vi "Waveform Channel Selection.vi"() -> ()   [LabVIEW 2015]
uses:
  NationalInstruments.VeriStand.SystemDefinitionAPI
  NationalInstruments.VeriStand.SystemStorage
  NationalInstruments.VeriStand
panel:
  in  "Commit Waveforms":bool
  in  "path":path=path "C:/Users/Public/Documents/National Instruments/NI VeriStand 2015/Examples/Stimulus Profile/Engine Demo/Engine Demo.nivssdf"
  in  "Stop Button":bool
  in  "Waveforms to Process":i32(listbox)
  in  "Available Unused Waveforms":i32(listbox)
  in  "Waveform Task":u16(ring) items=["Waveform1"=11, "Waveform2"=15]
  in  "Remove Channel":bool
  in  "Add Channel":bool
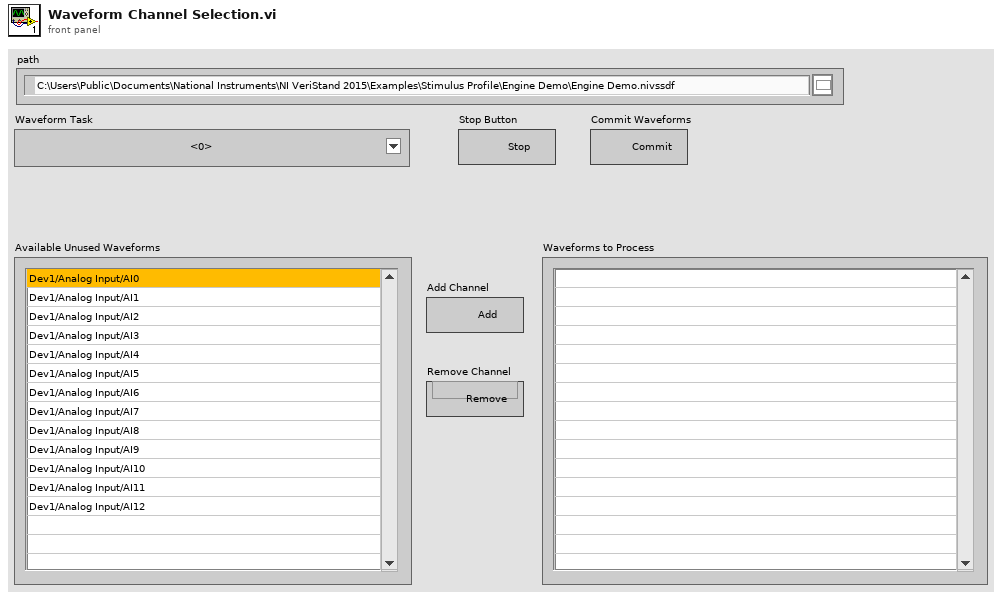
[diagram p1: front panel]
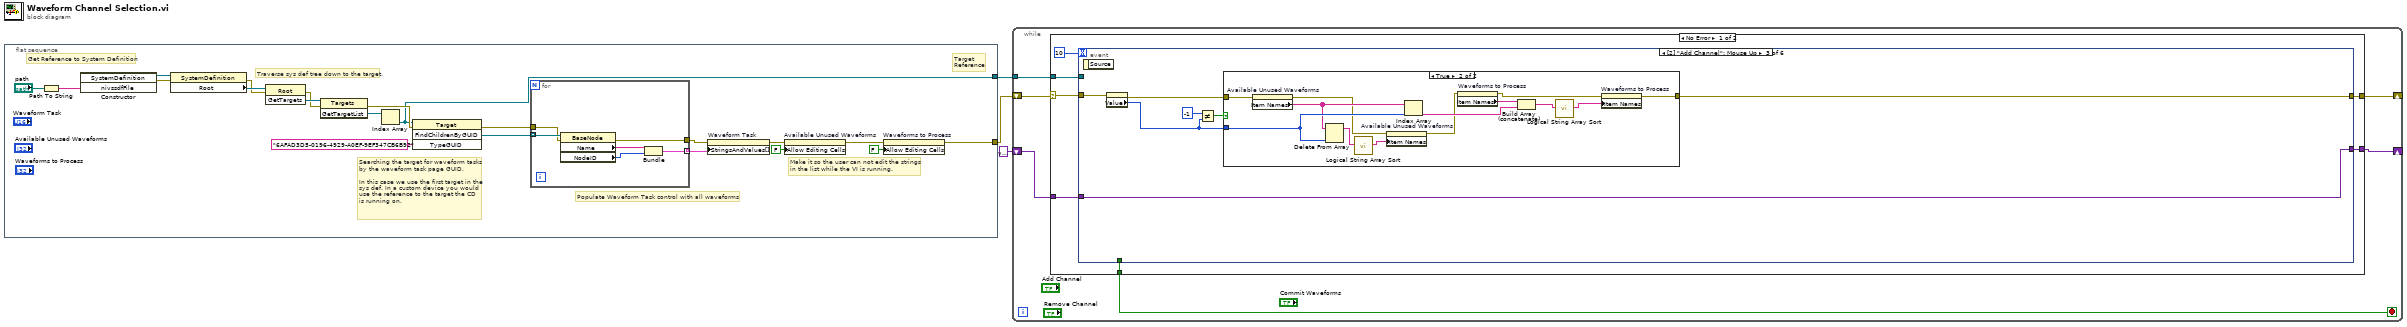
[diagram p0: block diagram]
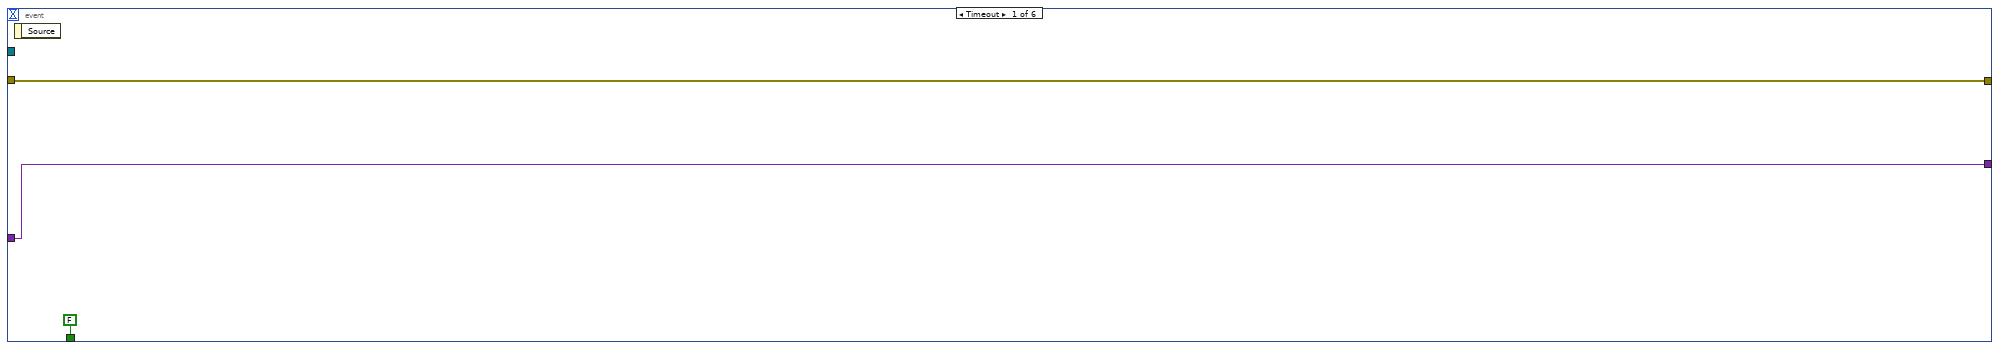
[diagram p2: hidden frame]
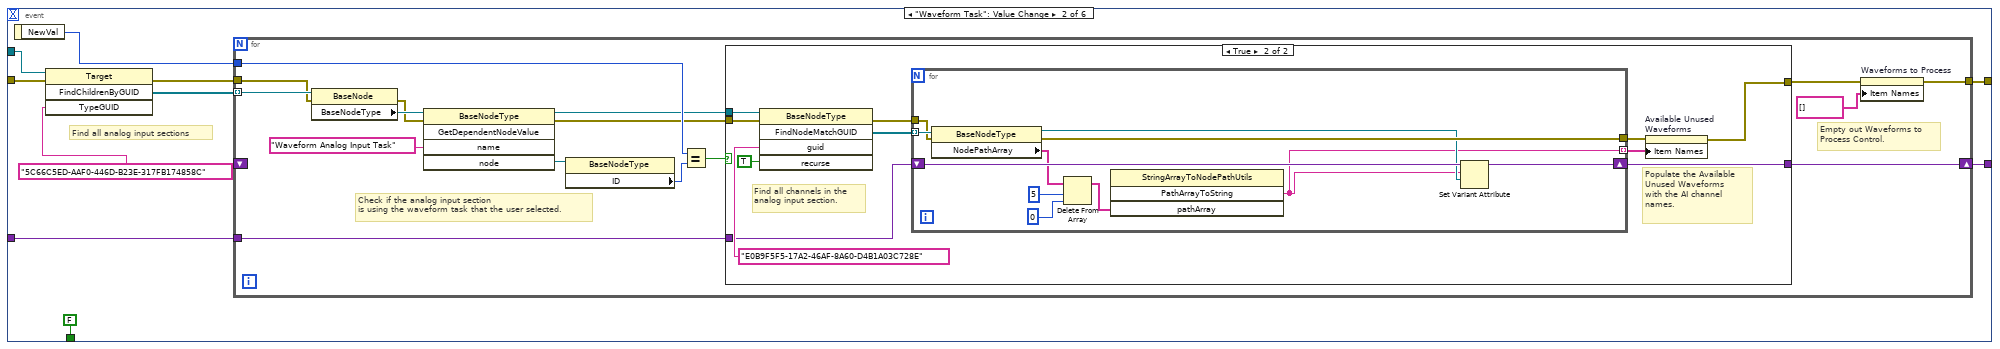
[diagram p3: hidden frame]
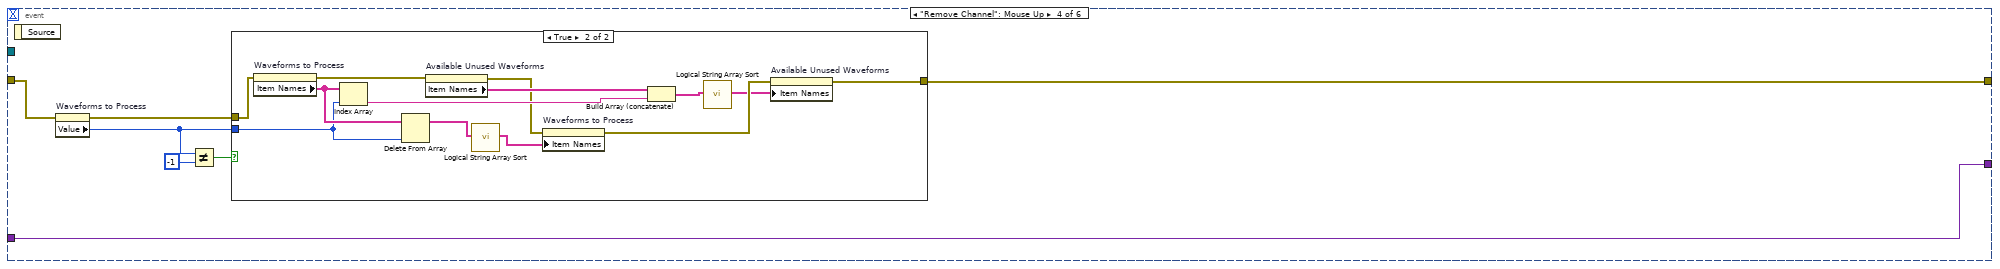
[diagram p6: hidden frame]
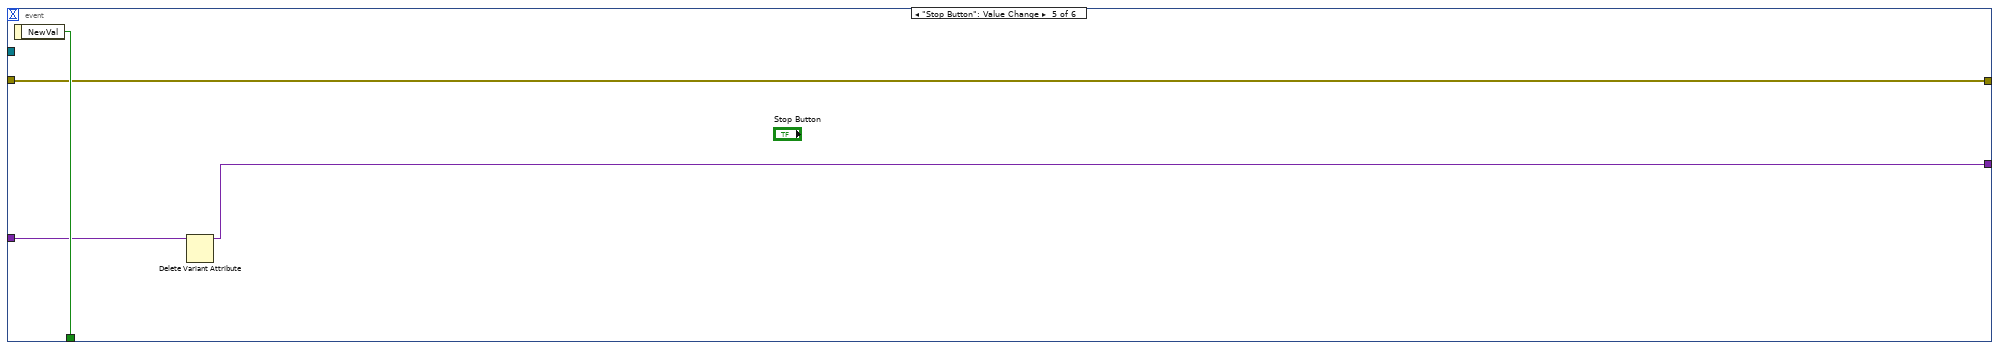
[diagram p8: hidden frame]
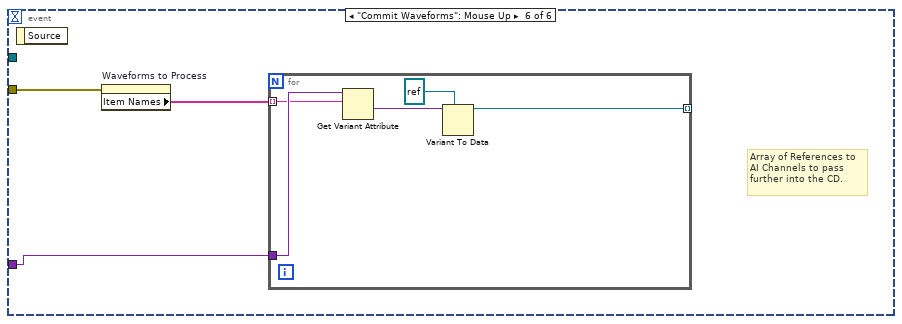
[diagram p9: hidden frame]
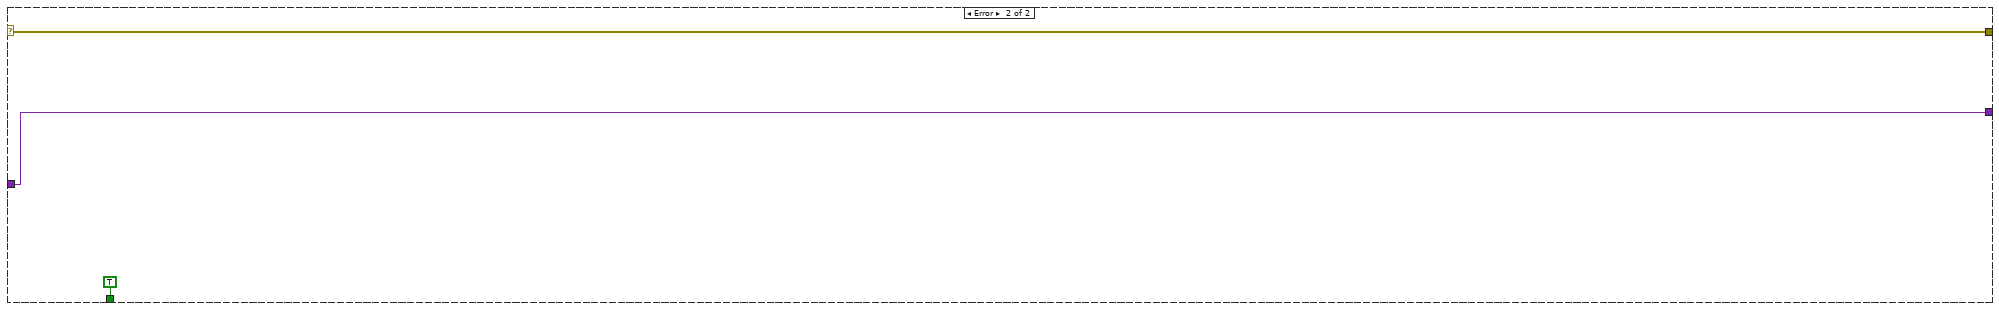
[diagram p10: hidden frame]
diagram:
  n1 = flat-sequence {
    tunnel: [w6] -> w2
    tunnel: [w9] -> w3
    frame #0 {
      # "Target\nReference"
      # "Make it so the user can not edit the strings\nin the list while the VI is running."
      # "Populate Waveform Task control with all waveforms"
      # "Traverse sys def tree down to the target."
      # "Get Reference to System Definition"
      # "Searching the target for waveform tasks\nby the waveform task page GUID.\n\nIn this case we use the first target in the \nsys def. In a custom device you would\nuse the reference to the target the CD\nis running on."
      n2 = Path To String(path="path") -> (string=w24:string)
      n3 = constructor class="SystemDefinition"("nivssdfFile"=w24) -> (reference out=w22:refnum<k24>, error out=w16:errorcluster)  [unwired: 3 in, 2 out]
      n4 = property class="SystemDefinition"(reference=w22, error in=w16) -> (error out=w15:errorcluster, "Root"=w21:refnum<k24>)  [unwired: 1 out]
      n5 = invoke class="Root" method="GetTargets"(reference=w21, error in=w15) -> (error out=w14:errorcluster, "GetTargets"=w20:refnum<k24>)  [unwired: 1 in, 1 out]
      n6 = invoke class="Targets" method="GetTargetList"(reference=w20, error in=w14) -> (error out=w13:errorcluster, "GetTargetList"=w19:refnum<k24>[])  [unwired: 1 in, 1 out]
      n7 = Index Array(array=w19) -> (element=w9:refnum<k24>)  [unwired: 1 in]
      n8 = invoke class="Target" method="FindChildrenByGUID"(reference=w9, error in=w13, "TypeGUID"="6AFAD3D5-0196-4929-A0EF-9EF347CB6B92") -> (error out=w12:errorcluster, "FindChildrenByGUID"=w17:refnum<k24>[])  [unwired: 1 in, 2 out]
      n9 = for {
        tunnel: w17 -> [w30] mode=indexing
        tunnel: [w27] -> w11 mode=indexing
        tunnel: w12 -> [w26]
        tunnel: [w25] -> w10
        n10 = property class="BaseNode"(reference=w30, error in=w26) -> (error out=w25:errorcluster, "Name"=w29:string, "NodeID"=w28:u64)  [unwired: 1 out]
        n11 = Bundle("Name"=w29, "NodeID"=w28) -> (w27:cluster{"Name":string, "NodeID":u64})  [unwired: 1 in]
      }
      n12 = property on="Waveform Task" class="Ring (strict)"(error in=w10, "StringsAndValues[]"=w11) -> (error out=w8:errorcluster)  [unwired: 1 in, 1 out]
      n13 = property on="Available Unused Waveforms" class="LstBox (strict)"(error in=w8, "Allow Editing Cells"=FALSE) -> (error out=w7:errorcluster)  [unwired: 1 in, 1 out]
      n14 = property on="Waveforms to Process" class="LstBox (strict)"(error in=w7, "Allow Editing Cells"=FALSE) -> (error out=w6:errorcluster)  [unwired: 1 in, 1 out]
    }
  }
  n15 = while {
    tunnel: w3 -> [w36]
    shift-right: [w34] -> _
    shift-left: w2 -> [w33]
    shift-right: [w31] -> _
    shift-left: variant -> [w32]
    stop <- w35 stop-if-true
    n16 = case shown="No Error" w33 {
      selector: w33 -> [w40 w151]
      tunnel: w36 -> [w42 _]
      tunnel: [w41 TRUE ("NewVal")] -> w35
      tunnel: [w39 w151] -> w34
      tunnel: [w38 w152] -> w31
      tunnel: w32 -> [w37 w152]
      frame No Error {
        n17 = event shown="[2] \"Add Channel\": Mouse Up" {
          selector: _ -> [_ _ _ _ _ _]
          dyn-events: _ -> [_ _ _ _ _ _]
          timeout: 10 -> [_ _ _ _ _ _]
          tunnel: w42 -> [_ w56 _ _ _ _]
          tunnel: [FALSE ("NewVal") FALSE ("NewVal") _ _ w142 _] -> w41
          tunnel: w40 -> [w44 w51 w102 w124 w139 w145]
          tunnel: [w44 w49 w100 w121 w139 _] -> w39
          tunnel: [w45 w48 w101 w122 w140 _] -> w38
          tunnel: w37 -> [w45 w47 w101 w122 w141 w143]
          event Timeout {
            n18 = event-data() -> ()  [unwired: 1 in, 1 out]
          }
          event "Waveform Task": Value Change {
            # "Find all analog input sections"
            n19 = event-data() -> ("NewVal"=w53:u16)  [unwired: 1 in]
            n20 = invoke class="Target" method="FindChildrenByGUID"(reference=w56, error in=w51, "TypeGUID"="5C66C5ED-AAF0-446D-B23E-317FB174858C") -> (error out=w50:errorcluster, "FindChildrenByGUID"=w54:refnum<k24>[])  [unwired: 1 in, 2 out]
            n21 = for {
              tunnel: w54 -> [w72] mode=indexing
              tunnel: w53 -> [w67]
              tunnel: w50 -> [w64]
              tunnel: [w59] -> w49
              shift-right: [w58] -> w48
              shift-left: _ -> [_]
              tunnel: w47 -> [w57]
              # "Empty out Waveforms to\nProcess Control."
              # "Check if the analog input section\nis using the waveform task that the user selected."
              n22 = property class="BaseNode"(reference=w72, error in=w64) -> (error out=w63:errorcluster, "BaseNodeType"=w71:refnum<k24>)  [unwired: 1 out]
              n23 = invoke class="BaseNodeType" method="GetDependentNodeValue"(reference=w71, error in=w63, "name"="Waveform Analog Input Task") -> (reference out=w65:refnum<k24>, error out=w62:errorcluster, "node"=w69:refnum<k24>)  [unwired: 2 in, 2 out]
              n24 = property class="BaseNodeType"(reference=w69) -> ("ID"=w68:u64)  [unwired: 1 in, 2 out]
              n25 = Equal?(x=w67, y=w68) -> (x = y?=w66:bool)
              n26 = case shown="True" w66 {
                tunnel: w65 -> [_ w85]
                tunnel: w62 -> [w74 w80]
                tunnel: [w74 w77] -> w60
                tunnel: [w73 w76] -> w58
                tunnel: w57 -> [w73 w75]
                frame False {
                }
                frame True {
                  # "Populate the Available\nUnused Waveforms \nwith the AI channel\nnames."
                  # "Find all channels in the\nanalog input section."
                  n27 = invoke class="BaseNodeType" method="FindNodeMatchGUID"(reference=w85, error in=w80, "guid"="E0B9F5F5-17A2-46AF-8A60-D4B1A03C728E", "recurse"=TRUE) -> (error out=w79:errorcluster, "FindNodeMatchGUID"=w82:refnum<k24>[])  [unwired: 1 in, 3 out]
                  n28 = for {
                    tunnel: w82 -> [w96] mode=indexing
                    tunnel: [w86] -> w81 mode=indexing
                    tunnel: w79 -> [w95]
                    tunnel: [w94] -> w78
                    shift-right: [w93] -> w76
                    shift-left: w75 -> [w92]
                    n29 = property class="BaseNodeType"(reference=w96, error in=w95) -> (reference out=w91:refnum<k24>, error out=w94:errorcluster, "NodePathArray"=w90:string[])
                    n30 = Delete From Array(array=w90, length=5, index=0) -> (array with subset deleted=w87:string[])  [unwired: 1 out]
                    n31 = invoke class="StringArrayToNodePathUtils" method="PathArrayToString"("pathArray"=w87) -> ("PathArrayToString"=w86:string)  [unwired: 3 in, 3 out]
                    n32 = Set Variant Attribute(Variant=w92, name=w86, value=w91) -> (Variant out=w93:variant)  [unwired: 1 in, 2 out]
                  }
                  n33 = property on="Available Unused Waveforms" class="LstBox (strict)"(error in=w78, "Item Names"=w81) -> (error out=w77:errorcluster)  [unwired: 1 in, 1 out]
                }
              }
              n34 = property on="Waveforms to Process" class="LstBox (strict)"(error in=w60, "Item Names"=string[] []) -> (error out=w59:errorcluster)  [unwired: 1 in, 1 out]
            }
          }
          event "Add Channel": Mouse Up {
            n35 = event-data() -> ()  [unwired: 1 in, 1 out]
            n36 = property on="Available Unused Waveforms" class="LstBox (strict)"(error in=w102) -> (error out=w103:errorcluster, "Value"=w98:i32)  [unwired: 1 in, 1 out]
            n37 = Not Equal?(x=-1, y=w98) -> (x != y?=w99:bool)
            n38 = case shown="True" w99 {
              tunnel: w103 -> [w104 w117]
              tunnel: w98 -> [_ w114]
              tunnel: [w104 w109] -> w100
              frame False {
              }
              frame True {
                n39 = property on="Available Unused Waveforms" class="LstBox (strict)"(error in=w117) -> (error out=w112:errorcluster, "Item Names"=w113:string[])  [unwired: 1 in, 1 out]
                n40 = Delete From Array(array=w113, index=w114) -> (array with subset deleted=w108:string[])  [unwired: 1 in, 1 out]
                n41 = call "Logical String Array Sort.vi"("Unsorted List"=w108) -> ("Sorted List"=w107:string[])  [unwired: 18 in]
                n42 = property on="Available Unused Waveforms" class="LstBox (strict)"(error in=w112, "Item Names"=w107) -> (error out=w111:errorcluster)  [unwired: 1 in, 1 out]
                n43 = Index Array(array=w113, index=w114) -> (element=w115:string)
                n44 = property on="Waveforms to Process" class="LstBox (strict)"(error in=w111) -> (error out=w110:errorcluster, "Item Names"=w116:string[])  [unwired: 1 in, 1 out]
                n45 = Build Array (concatenate)(w116, w115) -> (w106:string[])
                n46 = call "Logical String Array Sort.vi"("Unsorted List"=w106) -> ("Sorted List"=w105:string[])  [unwired: 18 in]
                n47 = property on="Waveforms to Process" class="LstBox (strict)"(error in=w110, "Item Names"=w105) -> (error out=w109:errorcluster)  [unwired: 1 in, 1 out]
              }
            }
          }
          event "Remove Channel": Mouse Up {
            n48 = event-data() -> ()  [unwired: 1 in, 1 out]
            n49 = property on="Waveforms to Process" class="LstBox (strict)"(error in=w124) -> (error out=w123:errorcluster, "Value"=w119:i32)  [unwired: 1 in, 1 out]
            n50 = Not Equal?(x=w119, y=-1) -> (x != y?=w120:bool)
            n51 = case shown="True" w120 {
              tunnel: w123 -> [w125 w138]
              tunnel: w119 -> [_ w134]
              tunnel: [w125 w130] -> w121
              frame False {
              }
              frame True {
                n52 = property on="Waveforms to Process" class="LstBox (strict)"(error in=w138) -> (error out=w133:errorcluster, "Item Names"=w135:string[])  [unwired: 1 in, 1 out]
                n53 = Index Array(array=w135, index=w134) -> (element=w136:string)
                n54 = Delete From Array(array=w135, index=w134) -> (array with subset deleted=w129:string[])  [unwired: 1 in, 1 out]
                n55 = property on="Available Unused Waveforms" class="LstBox (strict)"(error in=w133) -> (error out=w132:errorcluster, "Item Names"=w137:string[])  [unwired: 1 in, 1 out]
                n56 = call "Logical String Array Sort.vi"("Unsorted List"=w129) -> ("Sorted List"=w128:string[])  [unwired: 18 in]
                n57 = property on="Waveforms to Process" class="LstBox (strict)"(error in=w132, "Item Names"=w128) -> (error out=w131:errorcluster)  [unwired: 1 in, 1 out]
                n58 = Build Array (concatenate)(w137, w136) -> (w127:string[])
                n59 = call "Logical String Array Sort.vi"("Unsorted List"=w127) -> ("Sorted List"=w126:string[])  [unwired: 18 in]
                n60 = property on="Available Unused Waveforms" class="LstBox (strict)"(error in=w131, "Item Names"=w126) -> (error out=w130:errorcluster)  [unwired: 1 in, 1 out]
              }
            }
          }
          event "Stop Button": Value Change {
            n61 = event-data() -> ("NewVal"=w142:bool)  [unwired: 1 in]
            n62 = Delete Variant Attribute(7:w141) -> (3:w140:variant)  [unwired: 2 in, 2 out]
          }
          event "Commit Waveforms": Mouse Up {
            # "Array of References to\nAI Channels to pass \nfurther into the CD."
            n63 = event-data() -> ()  [unwired: 1 in, 1 out]
            n64 = property on="Waveforms to Process" class="LstBox (strict)"(error in=w145) -> ("Item Names"=w144:string[])  [unwired: 1 in, 2 out]
            n65 = for {
              tunnel: w144 -> [w149] mode=indexing
              tunnel: w143 -> [w150]
              tunnel: [w146] -> _ mode=indexing
              n66 = Get Variant Attribute(Variant=w150, name=w149) -> (value=w148:variant)  [unwired: 2 in, 3 out]
              n67 = Variant To Data(type=refnum<k24> refnum ("reference out"), Variant=w148) -> (data=w146:refnum<k24>)  [unwired: 1 in, 1 out]
            }
          }
        }
      }
      frame Error {
      }
    }
  }
